vi "EloMec Tester.vi"() -> ()   [LabVIEW 2021]
uses:
  Communication_class/Paths/Convert AI Robot to Robot Command Folder/grSim/grSim Robot Command.ctl
  Communication_class/feedbackData.ctl
  <vilib>/Instr/_visa.llb/VISA Configure Serial Port (Instr).vi
  Communication_class/Communication.lvclass
panel:
  in  "Modo":T1(ring)
  out "Battery":sgl(graph)
  in  "Feedback ID":u32
  out "Space":bool
  out "kickCharged":bool
  out "hasBall":bool
  out "E":bool
  out "Q":bool
  in  "Keyboard":bool=TRUE
  out "A":bool
  out "D":bool
  out "S":bool
  out "W":bool
  in  "Zero":bool
  out "Waveform Chart":T2(graph)
  out "FeedbackData":T3 {"status" format="%08x"}
  in  "FIRASim?":bool
  in  "IDs":u32[](array[numeric])=[0, 1, 2, 3, 4, 5, 6]
  out "Output Array":T4[](array[typedef])
  in  "chip kick":bool
  in  "kickspeedz":sgl=100.0
  in  "drible":bool
  in  "velangular":sgl
  in  "velnormal":sgl
  in  "veltangent":sgl
  in  "kick":bool
  in  "kickspeedx":sgl=100.0
  out "Numeric 2":u32
  out "String":string
  out "return count":u32
  in  "stop":bool
  out "string":string
  out "error out":errorcluster
  in  "termination char\n(0xA = '\\n' = LF)":u8=10 format="%.0x"
  in  "VISA resource name":refnum<visa-resource-name>
  in  "Serial Settings":T5={"baud rate"=9600, "data bits"=8, "parity"=enum."None", "stop bits"=10, "flow control"=0} {"flow control" items=["None"=0, "XON/XOFF"=1, "RTS/CTS"=2, "DTR/DSR"=4]; "stop bits" items=["1"=10, "1.5"=15, "2.0"=20]; "data bits" min=5 max=8 step=1; "baud rate" items=["75"=75, "110"=110, "134"=134, "150"=150, "300"=300, "600"=600, "1200"=1200, "1800"=1800, "2400"=2400, "4800"=4800, "7200"=7200, "9600"=9600, "14400"=14400, "19200"=19200, "28800"=28800, "38400"=38400, "56000"=56000, "57600"=57600, "115200"=115200, "128000"=128000, "230400"=230400]}
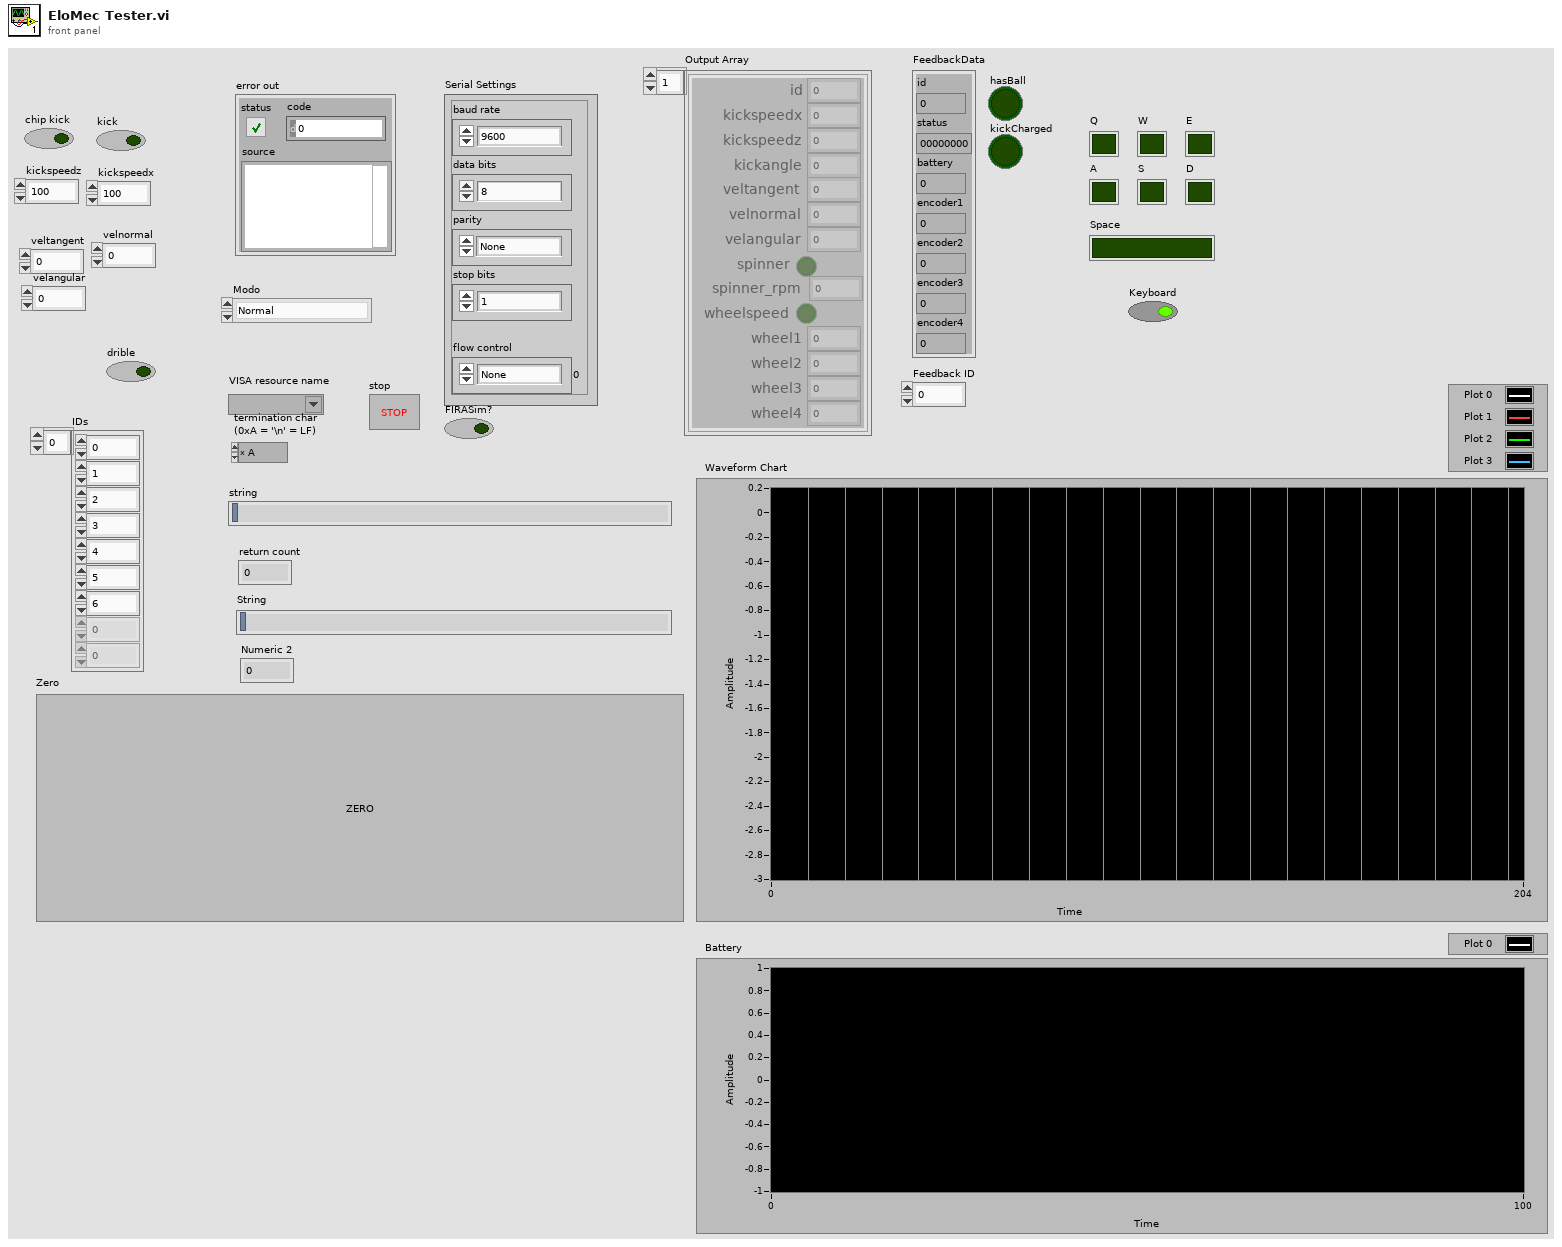
[diagram p1: front panel]
types:
  T1 = enum16{"Normal", "Rampa invertida", "Teste de engrenagem", "Rampa"}
  T2 = cluster{"[0]":sgl, "[1]":sgl, "[2]":sgl, "[3]":sgl, "[4]":sgl, "[5]":sgl, "[6]":sgl, "[7]":sgl, "[8]":sgl}
  T3 = typedef "feedbackData.ctl" = cluster{"id":u32, "status":u32, "battery":sgl, "encoder1":sgl, "encoder2":sgl, "encoder3":sgl, "encoder4":sgl}
  T4 = typedef "grSim Robot Command.ctl" = cluster{"id":u32, "kickspeedx":sgl, "kickspeedz":sgl, "veltangent":sgl, "velnormal":sgl, "velangular":sgl, "spinner":bool, "wheelspeed":bool, "wheel1":sgl, "wheel2":sgl, "wheel3":sgl, "wheel4":sgl, "kickangle":sgl, "spinner_rpm":sgl}
  T5 = cluster{"baud rate":u32, "data bits":u16, "parity":enum16{"None", "Odd", "Even", "Mark", "Space"}, "stop bits":u16, "flow control":u16}
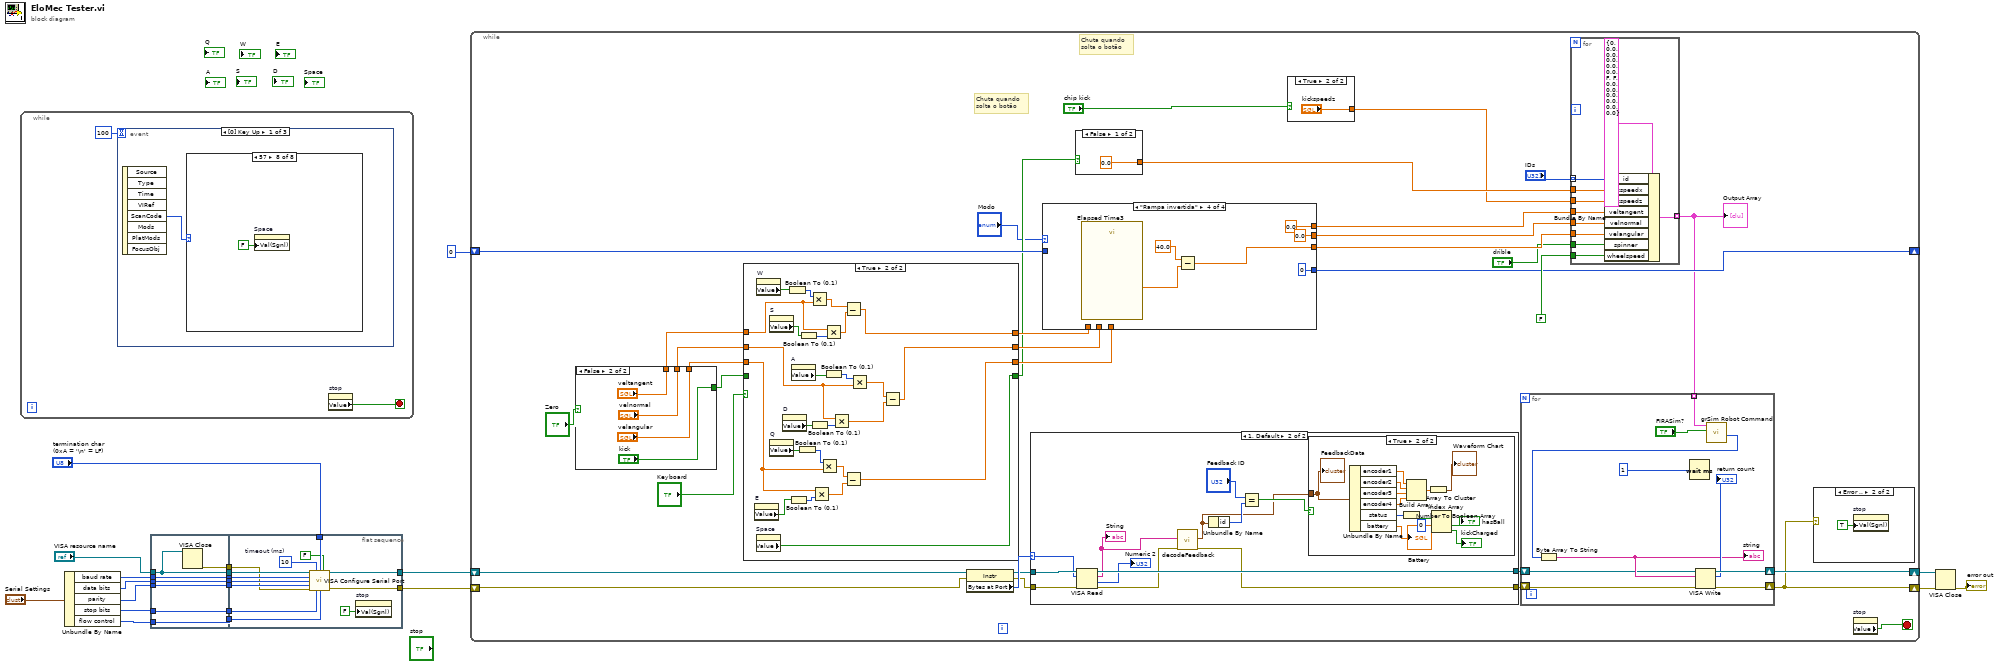
[diagram p0: block diagram]
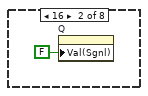
[diagram p3: hidden frame]
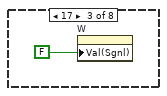
[diagram p4: hidden frame]
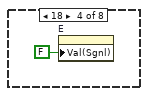
[diagram p5: hidden frame]
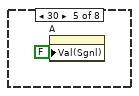
[diagram p6: hidden frame]
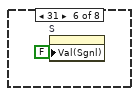
[diagram p7: hidden frame]
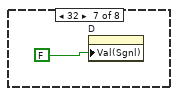
[diagram p8: hidden frame]
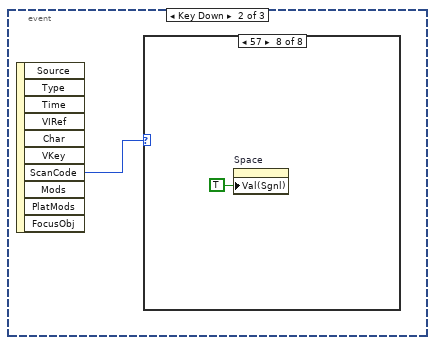
[diagram p9: hidden frame]
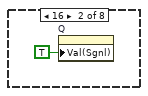
[diagram p11: hidden frame]
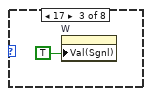
[diagram p12: hidden frame]
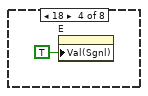
[diagram p13: hidden frame]
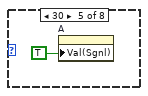
[diagram p14: hidden frame]
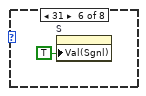
[diagram p15: hidden frame]
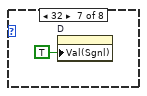
[diagram p16: hidden frame]
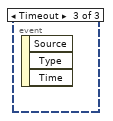
[diagram p17: hidden frame]
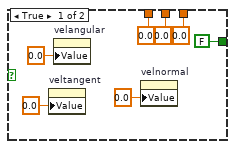
[diagram p20: hidden frame]
diagram:
  n1 = while {
    stop <- w23 stop-if-true
    n2 = event shown="[0] Key Up" {
      selector: _ -> [_ _ _]
      dyn-events: _ -> [_ _ _]
      timeout: 100 -> [_ _ _]
      event Key Up {
        n3 = event-data() -> ("ScanCode"=w24:i16)  [unwired: 1 in, 7 out]
        n4 = case shown="57" w24 {
          frame Default {
          }
          frame 16 {
            n5 = property on="Q" class="Bool (strict)"("Val(Sgnl)"=FALSE ("Value (Signaling)")) -> ()  [unwired: 2 in, 2 out]
          }
          frame 17 {
            n6 = property on="W" class="Bool (strict)"("Val(Sgnl)"=FALSE ("W")) -> ()  [unwired: 2 in, 2 out]
          }
          frame 18 {
            n7 = property on="E" class="Bool (strict)"("Val(Sgnl)"=FALSE ("Value (Signaling)")) -> ()  [unwired: 2 in, 2 out]
          }
          frame 30 {
            n8 = property on="A" class="Bool (strict)"("Val(Sgnl)"=FALSE ("A")) -> ()  [unwired: 2 in, 2 out]
          }
          frame 31 {
            n9 = property on="S" class="Bool (strict)"("Val(Sgnl)"=FALSE ("S")) -> ()  [unwired: 2 in, 2 out]
          }
          frame 32 {
            n10 = property on="D" class="Bool (strict)"("Val(Sgnl)"=FALSE ("D")) -> ()  [unwired: 2 in, 2 out]
          }
          frame 57 {
            n11 = property on="Space" class="Bool (strict)"("Val(Sgnl)"=FALSE ("Value (Signaling)")) -> ()  [unwired: 2 in, 2 out]
          }
        }
      }
      event Key Down {
        n12 = event-data() -> ("ScanCode"=w32:i16)  [unwired: 1 in, 9 out]
        n13 = case shown="57" w32 {
          frame Default {
          }
          frame 16 {
            n14 = property on="Q" class="Bool (strict)"("Val(Sgnl)"=TRUE ("Value (Signaling)")) -> ()  [unwired: 2 in, 2 out]
          }
          frame 17 {
            n15 = property on="W" class="Bool (strict)"("Val(Sgnl)"=TRUE) -> ()  [unwired: 2 in, 2 out]
          }
          frame 18 {
            n16 = property on="E" class="Bool (strict)"("Val(Sgnl)"=TRUE ("Value (Signaling)")) -> ()  [unwired: 2 in, 2 out]
          }
          frame 30 {
            n17 = property on="A" class="Bool (strict)"("Val(Sgnl)"=TRUE) -> ()  [unwired: 2 in, 2 out]
          }
          frame 31 {
            n18 = property on="S" class="Bool (strict)"("Val(Sgnl)"=TRUE) -> ()  [unwired: 2 in, 2 out]
          }
          frame 32 {
            n19 = property on="D" class="Bool (strict)"("Val(Sgnl)"=TRUE) -> ()  [unwired: 2 in, 2 out]
          }
          frame 57 {
            n20 = property on="Space" class="Bool (strict)"("Val(Sgnl)"=TRUE ("Value (Signaling)")) -> ()  [unwired: 2 in, 2 out]
          }
        }
      }
      event Timeout {
        n21 = event-data() -> ()  [unwired: 1 in, 3 out]
      }
    }
    n22 = property on="stop" class="Bool (strict)"() -> ("Value"=w23:bool)  [unwired: 2 in, 2 out]
  }
  n23 = Unbundle By Name("Serial Settings") -> ("baud rate"=w20:u32, "data bits"=w19:u16, "parity"=w18:enum16{"None", "Odd", "Even", "Mark", "Space"}, "stop bits"=w17:u16, "flow control"=w16:u16)
  n24 = flat-sequence {
    tunnel: "VISA resource name" -> [w41]
    tunnel: w16 -> [w42]
    tunnel: w17 -> [w43]
    tunnel: w18 -> [w44]
    tunnel: w19 -> [w45]
    tunnel: w20 -> [w46]
    tunnel: [w46] -> w8
    tunnel: [w45] -> w7
    tunnel: [w44] -> w6
    tunnel: [w43] -> w5
    tunnel: [w42] -> w4
    tunnel: [w41] -> w3
    tunnel: [w40] -> w2
    tunnel: "termination char\n(0xA = '\\n' = LF)" -> [w53]
    tunnel: [w51] -> w13
    tunnel: [w50] -> w11
    tunnel: w8 -> [w59]
    tunnel: w7 -> [w58]
    tunnel: w6 -> [w57]
    tunnel: w5 -> [w56]
    tunnel: w4 -> [w55]
    tunnel: w3 -> [w54]
    tunnel: w2 -> [w48]
    frame #0 {
      n25 = VISA Close(VISA resource name=w41) -> (error out=w40:errorcluster)  [unwired: 1 in]
    }
    frame #1 {
      w49 = u32 10  # timeout (ms)
      n26 = call-poly "VISA Configure Serial Port"("VISA resource name"=w54, "timeout (10sec)"=w49, "termination char\n(0xA = '\\n' = LF)"=w53, "Enable Termination\nChar (T)"=FALSE ("Enable Termination\nChar (T)"), "baud rate (9600)"=w59, "data bits (8)"=w58, "parity (0:none)"=w57, "error in (no error)"=w48, "stop bits (10: 1 bit)"=w56, "flow control (0:none)"=w55) -> ("VISA resource name out"=w51:refnum<visa-resource-name>, "error out"=w50:errorcluster)  [unwired: 4 in]
      n27 = property on="stop" class="Bool (strict)"("Val(Sgnl)"=FALSE ("Value (Signaling)")) -> ()  [unwired: 2 in, 2 out]
    }
  }
  n28 = while {
    shift-right: [w92] -> w12
    shift-left: w13 -> [w88]
    shift-right: [w64] -> w10
    shift-left: w11 -> [w87]
    shift-right: [w77] -> _
    shift-left: 0 -> [w78]
    stop <- w65 stop-if-true
    # "Chuta quando \nsolta o botão"
    # "Chuta quando \nsolta o botão"
    n29 = case shown="False" "Zero" {
      tunnel: [sgl 0.0 ("veltangent") "veltangent"] -> w69
      tunnel: [sgl 0.0 ("velnormal") "velnormal"] -> w70
      tunnel: [sgl 0.0 ("velangular") "velangular"] -> w71
      tunnel: [FALSE ("kick") "kick"] -> w62
      frame True {
        n30 = property on="veltangent" class="DigNum (strict)"("Value"=sgl 0.0 ("veltangent")) -> ()  [unwired: 2 in, 2 out]
        n31 = property on="velangular" class="DigNum (strict)"("Value"=sgl 0.0 ("velangular")) -> ()  [unwired: 2 in, 2 out]
        n32 = property on="velnormal" class="DigNum (strict)"("Value"=sgl 0.0 ("velnormal")) -> ()  [unwired: 2 in, 2 out]
      }
      frame False {
      }
    }
    n33 = case shown="True" "Keyboard" {
      tunnel: w71 -> [w95 w117]
      tunnel: w70 -> [w96 w101]
      tunnel: w69 -> [w97 w110]
      tunnel: [w97 w107] -> w68
      tunnel: [w96 w99] -> w67
      tunnel: [w95 w115] -> w66
      tunnel: w62 -> [w94 _]
      tunnel: [w94 w98] -> w61
      frame False {
      }
      frame True {
        n34 = property on="E" class="Bool (strict)"() -> ("Value"=w121:bool)  [unwired: 2 in, 2 out]
        n35 = property on="Space" class="Bool (strict)"() -> ("Value"=w98:bool)  [unwired: 2 in, 2 out]
        n36 = property on="W" class="Bool (strict)"() -> ("Value"=w114:bool)  [unwired: 2 in, 2 out]
        n37 = property on="S" class="Bool (strict)"() -> ("Value"=w112:bool)  [unwired: 2 in, 2 out]
        n38 = property on="Q" class="Bool (strict)"() -> ("Value"=w122:bool)  [unwired: 2 in, 2 out]
        n39 = property on="D" class="Bool (strict)"() -> ("Value"=w103:bool)  [unwired: 2 in, 2 out]
        n40 = Boolean To (0,1)(Boolean=w114) -> (0, 1=w113:i16)
        n41 = Boolean To (0,1)(Boolean=w121) -> (0, 1=w118:i16)
        n42 = property on="A" class="Bool (strict)"() -> ("Value"=w106:bool)  [unwired: 2 in, 2 out]
        n43 = Boolean To (0,1)(Boolean=w122) -> (0, 1=w120:i16)
        n44 = Boolean To (0,1)(Boolean=w112) -> (0, 1=w111:i16)
        n45 = Multiply(x=w113, y=w110) -> (x*y=w109:sgl)
        n46 = Boolean To (0,1)(Boolean=w103) -> (0, 1=w102:i16)
        n47 = Multiply(x=w117, y=w118) -> (x*y=w116:sgl)
        n48 = Multiply(x=w120, y=w117) -> (x*y=w119:sgl)
        n49 = Boolean To (0,1)(Boolean=w106) -> (0, 1=w105:i16)
        n50 = Multiply(x=w110, y=w111) -> (x*y=w108:sgl)
        n51 = Multiply(x=w101, y=w102) -> (x*y=w100:sgl)
        n52 = Subtract(x=w109, y=w108) -> (x-y=w107:sgl)
        n53 = Subtract(x=w119, y=w116) -> (x-y=w115:sgl)
        n54 = Multiply(x=w105, y=w101) -> (x*y=w104:sgl)
        n55 = Subtract(x=w104, y=w100) -> (x-y=w99:sgl)
      }
    }
    n56 = property class="Instr"(reference=w88, error in=w87) -> (reference out=w84:refnum<visa-resource-name>, error out=w85:errorcluster, "Bytes at Port"=w86:u32)
    n57 = case shown="1, Default" w86 {
      selector: w86 -> [_ w197]
      tunnel: w85 -> [w188 w201]
      tunnel: [w188 w194] -> w90
      tunnel: w84 -> [w189 w200]
      tunnel: [w189 w199] -> w89
      frame 0 {
      }
      frame 1, Default {
        n58 = VISA Read(VISA resource name=w200, byte count=w197, error in (no error)=w201) -> (VISA resource name out=w199:refnum<visa-resource-name>, read buffer=w196:string, return count=→"Numeric 2":u32, error out=w195:errorcluster)
        "String" <- w196
        n59 = call "decodeFeedback.vi"("error in (no error)"=w195, "String"=w196) -> ("error out"=w194:errorcluster, "FeedbackData"=w190:T3)  [unwired: 7 in, 1 out]
        n60 = Unbundle By Name(w190) -> ("id"=w192:u32)
        n61 = Equal?(x="Feedback ID", y=w192) -> (x = y?=w191:bool)
        n62 = case shown="True" w191 {
          tunnel: w190 -> [_ w204]
          frame False {
          }
          frame True {
            n63 = Unbundle By Name(w204) -> ("encoder1"=w203:sgl, "encoder2"=w214:sgl, "encoder3"=w213:sgl, "encoder4"=w212:sgl, "status"=w209:u32, "battery"=→"Battery":sgl)
            n64 = Number To Boolean Array(number=w209) -> (Boolean array=w208:bool[])
            n65 = Build Array(w203, w214, w213, w212) -> (w211:sgl[])
            n66 = Array To Cluster(array=w211) -> (cluster=→"Waveform Chart":T2)
            n67 = Index Array(array=w208, index #1=0 ("index")) -> (element #1=→"hasBall":bool, element #2=→"kickCharged":bool)  [unwired: 1 in]
            "FeedbackData" <- w204
          }
        }
      }
    }
    n68 = case shown="\"Rampa invertida\"" "Modo" {
      tunnel: [w159 sgl 0.0 ("veltangent") sgl 0.0 ("veltangent") sgl 0.0 ("veltangent")] -> w82
      tunnel: w68 -> [w159 _ _ _]
      tunnel: [w158 w160 sgl 0.0 ("velnormal") sgl 0.0 ("velnormal")] -> w81
      tunnel: w67 -> [w158 w161 _ _]
      tunnel: w66 -> [w157 _ _ _]
      tunnel: [w157 sgl 0.0 ("velangular") w179 w183] -> w80
      tunnel: w78 -> [_ w166 _ _]
      tunnel: [0 w165 0 0] -> w77
      frame "Normal" {
      }
      frame "Teste de engrenagem" {
        n69 = call "Elapsed Time"() -> ("Time has Elapsed"=w169:bool)  [unwired: 12 in, 7 out]
        n70 = case shown="False" w169 {
          tunnel: w166 -> [w173 w175]
          tunnel: [w173 w174] -> w165
          frame False {
          }
          frame True {
            n71 = Increment(x=w175) -> (x+1=w174:i32)
          }
        }
        n72 = Quotient & Remainder(x=w165, y=2) -> (x-y*floor(x/y)=w163:i32)  [unwired: 1 out]
        n73 = Equal To 0?(x=w163) -> (x = 0?=w162:bool)
        n74 = case shown="True" w162 {
          tunnel: w161 -> [w171 w172]
          tunnel: [w170 w172] -> w160
          frame False {
            n75 = Negate(x=w171) -> (-x=w170:sgl)
          }
          frame True {
          }
        }
      }
      frame "Rampa" {
        n76 = call "Elapsed Time2"() -> ("Elapsed Time (s)"=w179:dbl)  [unwired: 12 in, 7 out]
      }
      frame "Rampa invertida" {
        n77 = call "Elapsed Time3"() -> ("Elapsed Time (s)"=w184:dbl)  [unwired: 12 in, 7 out]
        n78 = Subtract(x=40.0, y=w184) -> (x-y=w183:dbl)
      }
    }
    n79 = case shown="False" w61 {
      tunnel: [sgl 0.0 ("kickspeedx") "kickspeedx"] -> w83
      frame False {
      }
      frame True {
      }
    }
    n80 = case shown="True" "chip kick" {
      tunnel: [sgl 0.0 ("kickspeedx") "kickspeedz"] -> w76
      frame False {
      }
      frame True {
      }
    }
    n81 = for {
      tunnel: FALSE -> [w153]
      tunnel: w83 -> [w152]
      tunnel: w82 -> [w151]
      tunnel: w81 -> [w150]
      tunnel: w80 -> [w149]
      tunnel: "drible" -> [w148]
      tunnel: w76 -> [w147]
      tunnel: [w146] -> w74 mode=indexing
      tunnel: "IDs" -> [w144] mode=indexing
      n82 = Bundle By Name(cluster=T4 {"id"=0, "kickspeedx"=0.0, "kickspeedz"=0.0, "veltangent"=0.0, "velnormal"=0.0, "velangular"=0.0, "spinner"=FALSE, "wheelspeed"=FALSE, "wheel1"=0.0, "wheel2"=0.0, "wheel3"=0.0, "wheel4"=0.0, "kickangle"=0.0, "spinner_rpm"=0.0} ("Robots"), "id"=w144, "kickspeedx"=w152, "kickspeedz"=w147, "veltangent"=w151, "velnormal"=w150, "velangular"=w149, "spinner"=w148, "wheelspeed"=w153) -> (w146:T4)
    }
    "Output Array" <- w74
    n83 = for {
      shift-right: [w141] -> w64
      shift-left: w90 -> [w137]
      shift-right: [w143] -> w92
      shift-left: w89 -> [w136]
      tunnel: w74 -> [w135] mode=indexing
      n84 = Wait (ms)(milliseconds to wait=u32 1) -> ()  [unwired: 1 out]
      n85 = call "grSim Robot Command.vi"("FIRASim?"="FIRASim?", "Robots"=w135) -> ("Array"=w138:u8[])  [unwired: 9 in]
      n86 = Byte Array To String(unsigned byte array=w138) -> (string=w139:string)
      "string" <- w139
      n87 = VISA Write(VISA resource name=w136, write buffer=w139, error in (no error)=w137) -> (VISA resource name out=w143:refnum<visa-resource-name>, return count=→"return count":u32, error out=w141:errorcluster)
    }
    n88 = case shown="Error .." w64 {
      frame No Error {
      }
      frame Error {
        n89 = property on="stop" class="Bool (strict)"("Val(Sgnl)"=TRUE ("Value (Signaling)")) -> ()  [unwired: 2 in, 2 out]
      }
    }
    n90 = property on="stop" class="Bool (strict)"() -> ("Value"=w65:bool)  [unwired: 2 in, 2 out]
  }
  n91 = VISA Close(VISA resource name=w12, error in (no error)=w10) -> (error out=→"error out":errorcluster)
